vi "Freeze value.vi"(9 "Freeze Value":bool=TRUE, 11 "input":dbl) -> (3 "output":dbl)   [LabVIEW 2019]
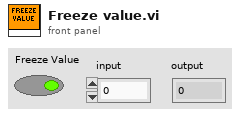
[diagram p1: front panel]
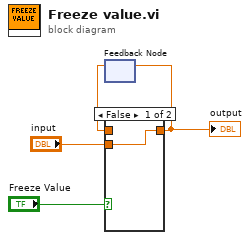
[diagram p0: block diagram]
diagram:
  n1 = feedback #1() -> (w4:dbl)  [unwired: 1 in]
  n2 = case shown="False" "Freeze Value" {
    tunnel: [w5 w6] -> w2
    tunnel: w4 -> [_ w6]
    tunnel: "input" -> [w5 _]
    frame False {
    }
    frame True {
    }
  }
  "output" <- w2
  n3 = feedback-in #1(w2) -> ()
